vi "Write Configuration Data.vi"(8 "error in":errorcluster, 10 "Configuration Settings":T1, 11 "File Path":path) -> (0 "error out":errorcluster)   [LabVIEW 2021]
uses:
  controls/Configuration Settings.ctl
  <vilib>/Utility/config.llb/Write Key (I32).vi
  <vilib>/Utility/config.llb/Write Key (Double).vi
  <vilib>/Utility/config.llb/Write Key (String).vi
  <vilib>/Utility/config.llb/NI_LVConfig.lvlib
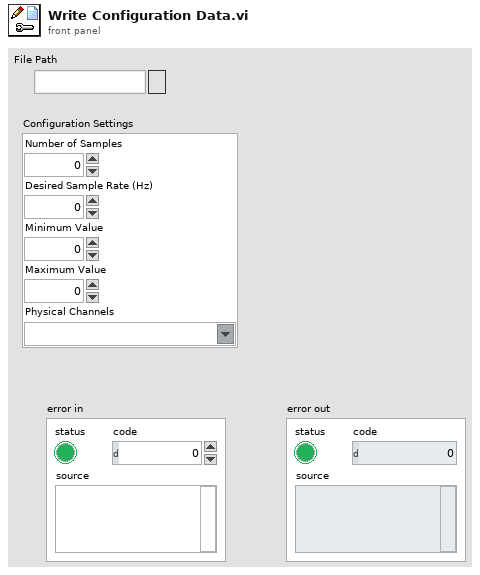
[diagram p1: front panel]
types:
  T1 = typedef "Configuration Settings.ctl" = cluster{"Number of Samples":i32, "Desired Sample Rate (Hz)":dbl, "Minimum Value":dbl, "Maximum Value":dbl, "Physical Channels":tag}
  T2 = typedef "NI_LVConfig.lvlib/Config Data RefNum.ctl" = refnum<k1>
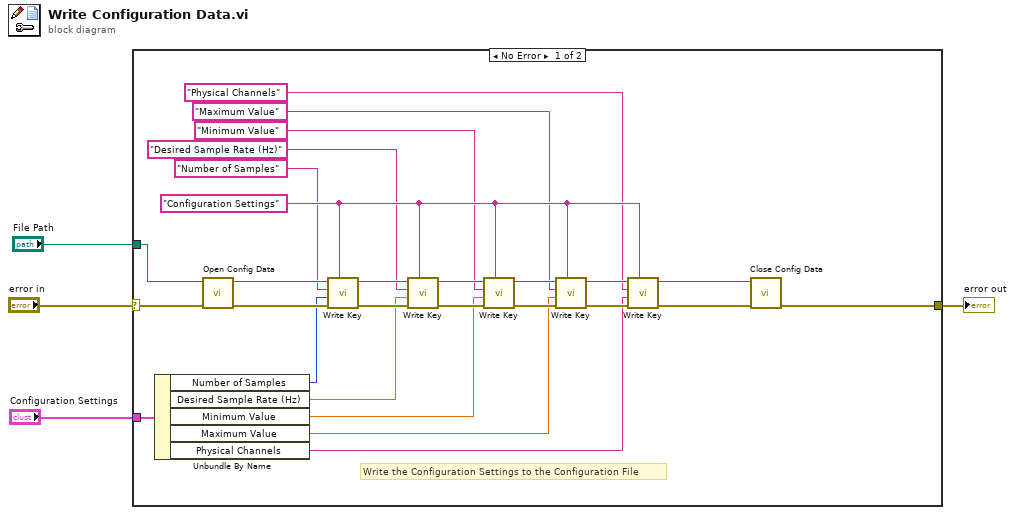
[diagram p0: block diagram]
diagram:
  n1 = case shown="No Error" "error in" {
    selector: "error in" -> [w31 w32]
    tunnel: [w24 w32] -> w3
    tunnel: "File Path" -> [w23 _]
    tunnel: "Configuration Settings" -> [w16 _]
    frame No Error {
      w11 = "Configuration Settings"
      # "Write the Configuration Settings to the Configuration File"
      n2 = Unbundle By Name(w16) -> ("Number of Samples"=w15:i32, "Desired Sample Rate (Hz)"=w14:dbl, "Minimum Value"=w13:dbl, "Maximum Value"=w6:dbl, "Physical Channels"=w12:tag)
      n3 = call <vilib>:"Open Config Data.vi"("error in (no error)"=w31, "configuration file path"=w23) -> ("error out"=w30:errorcluster, "refnum"=w22:T2)  [unwired: 7 in, 1 out]
      n4 = call-poly <vilib>:"Write Key.vi"("section"=w11, "error in (no error)"=w30, "value"=w15, "key"="Number of Samples", "refnum"=w22) -> ("error out"=w29:errorcluster, "refnum out"=w21:T2)  [unwired: 4 in, 1 out]
      n5 = call-poly <vilib>:"Write Key.vi"("section"=w11, "error in (no error)"=w29, "value"=w14, "key"="Desired Sample Rate (Hz)", "refnum"=w21) -> ("error out"=w28:errorcluster, "refnum out"=w20:T2)  [unwired: 4 in, 1 out]
      n6 = call-poly <vilib>:"Write Key.vi"("section"=w11, "error in (no error)"=w28, "value"=w13, "key"="Minimum Value", "refnum"=w20) -> ("error out"=w27:errorcluster, "refnum out"=w19:T2)  [unwired: 4 in, 1 out]
      n7 = call-poly <vilib>:"Write Key.vi"("section"=w11, "error in (no error)"=w27, "value"=w6, "key"="Maximum Value", "refnum"=w19) -> ("error out"=w26:errorcluster, "refnum out"=w18:T2)  [unwired: 4 in, 1 out]
      n8 = call-poly <vilib>:"Write Key.vi"("section"=w11, "error in (no error)"=w26, "value"=w12, "key"="Physical Channels", "refnum"=w18) -> ("error out"=w25:errorcluster, "refnum out"=w17:T2)  [unwired: 4 in, 1 out]
      n9 = call <vilib>:"Close Config Data.vi"("error in (no error)"=w25, "refnum"=w17) -> ("error out"=w24:errorcluster)  [unwired: 8 in, 1 out]
    }
    frame Error {
    }
  }
  "error out" <- w3
